vi "Process Outgoing Messages by Frame Type.vi"(0 "J1939 Cluster":T7, 5 "Output Array":T8[](array[typedef]) {"Identifier" format="%08x"}, 7 "Connection Refs":T1, 11 "error in":errorcluster) -> (4 "J1939 Cluster":T7, 13 "Message Errors":errorcluster, 15 "System Error":errorcluster)   [LabVIEW 2013, in "J1939 Addon Engine.lvlib"]
uses:
  Engine/J1939 Addon Engine.lvlib
  J1939 Utilities/Types/CAN Outgoing Message Cluster.ctl
  Types/Setup Information Cluster.ctl
  <vilib>/xnet/xnet.llb/XNET Frame CAN.ctl
  <vilib>/xnet/xnet.llb/XNET Frame Type CAN.ctl
  Types/TP List References.ctl
  Types/BAM Buffer Connections List_Ref.ctl
  Types/Connection Mode Generation Connection Ref.ctl
  Types/BAM Generation Connections List_Ref.ctl
  Types/Address Table Reference.ctl
  Types/RQST Lookup Table Reference.ctl
  Types/TP Connections List State.ctl
  BAM Generation Connections List_Actions.vi
  BAM Generation Create New TP Connection.vi
  Connection Mode Generation Connections List_Actions.vi
  Connection Mode Generation Search for Connection (Local Message).vi
  Connection Mode Generation Create New TP Connection.vi
  J1939 Utilities/Common Conversions.vi
  J1939 Utilities/SubVIs/Convert CAN Arb ID to J1939 ID.vi
  J1939 Utilities/Common Messages.vi
  J1939 Utilities/SubVIs/TP.CM BAM.vi
  J1939 Utilities/SubVIs/TP.DT.vi
  J1939 Utilities/SubVIs/TP.CM RTS.vi
  J1939 Utilities/SubVIs/Convert J1939 ID to CAN Arb ID.vi
  BAM Generation Search for Connection (Local Message).vi
  J1939 Utilities/J1939 Utilities.lvlib
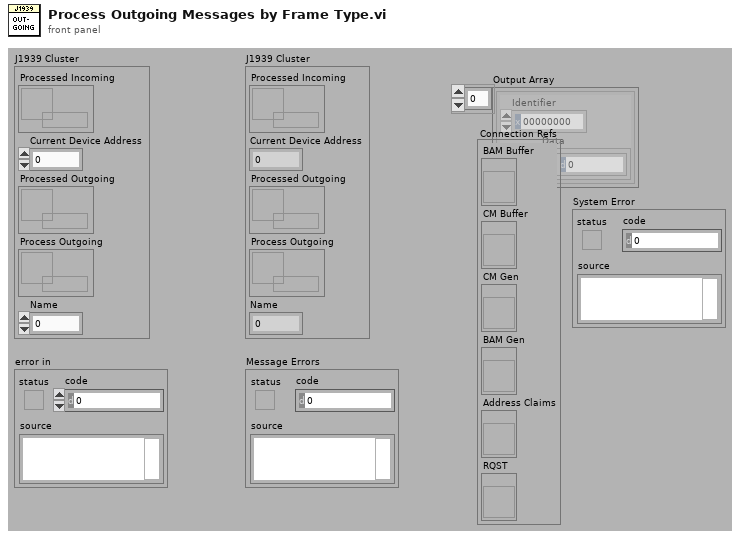
[diagram p1: front panel]
types:
  T1 = typedef "J1939 Addon Engine.lvlib/TP List References.ctl" = cluster{"BAM Buffer":T2, "CM Buffer":T2, "CM Gen":T3, "BAM Gen":T4, "Address Claims":T5, "RQST":T6}
  T2 = typedef "J1939 Addon Engine.lvlib/BAM Buffer Connections List_Ref.ctl" = refnum<vi>
  T3 = typedef "J1939 Addon Engine.lvlib/Connection Mode Generation Connection Ref.ctl" = refnum<vi>
  T4 = typedef "J1939 Addon Engine.lvlib/BAM Generation Connections List_Ref.ctl" = refnum<vi>
  T5 = typedef "J1939 Addon Engine.lvlib/Address Table Reference.ctl" = refnum<vi>
  T6 = typedef "J1939 Addon Engine.lvlib/RQST Lookup Table Reference.ctl" = refnum<vi>
  T7 = typedef "J1939 Addon Engine.lvlib/Setup Information Cluster.ctl" = cluster{"Processed Incoming":refnum<queue>, "Current Device Address":u8, "Processed Outgoing":refnum<queue>, "Process Outgoing":refnum<queue>, "Name":u64}
  T8 = typedef "J1939 Addon Shared.lvlib/J1939 Utilities.lvlib/CAN Outgoing Message Cluster.ctl" = cluster{"Identifier":u32, "Data":u8[]}
  T9 = typedef "J1939 Addon Engine.lvlib/TP Connections List State.ctl" = enum16{"Add", "Update", "Get", "Remove", "Initialize"}
  T10 = typedef "J1939 Addon Shared.lvlib/J1939 Utilities.lvlib/Outgoing Messages Frame Type.ctl" = enum16{"Standard Frame", "BAM", "Connection Mode"}
  T11 = typedef "J1939 Addon Engine.lvlib/BAM Generation Connection Cluster.ctl" = cluster{"Total Packets":u8, "Current Packet to Generate":u8, "Packets":T8[], "Previous Time Stamp":u32, "Total Bytes":u16, "Source Address":u8}
  T12 = typedef "J1939 Addon Engine.lvlib/Connection Mode Generation Connection Cluster.ctl" = cluster{"Total Packets":u8, "Current Packet to Generate":u8, "Packets":T8[], "Previous Time Stamp":u32, "Total Bytes":u16, "Packet Identifier [PDU S + SA]":u16, "Number of Packets to Generate":u8, "PGN":u32}
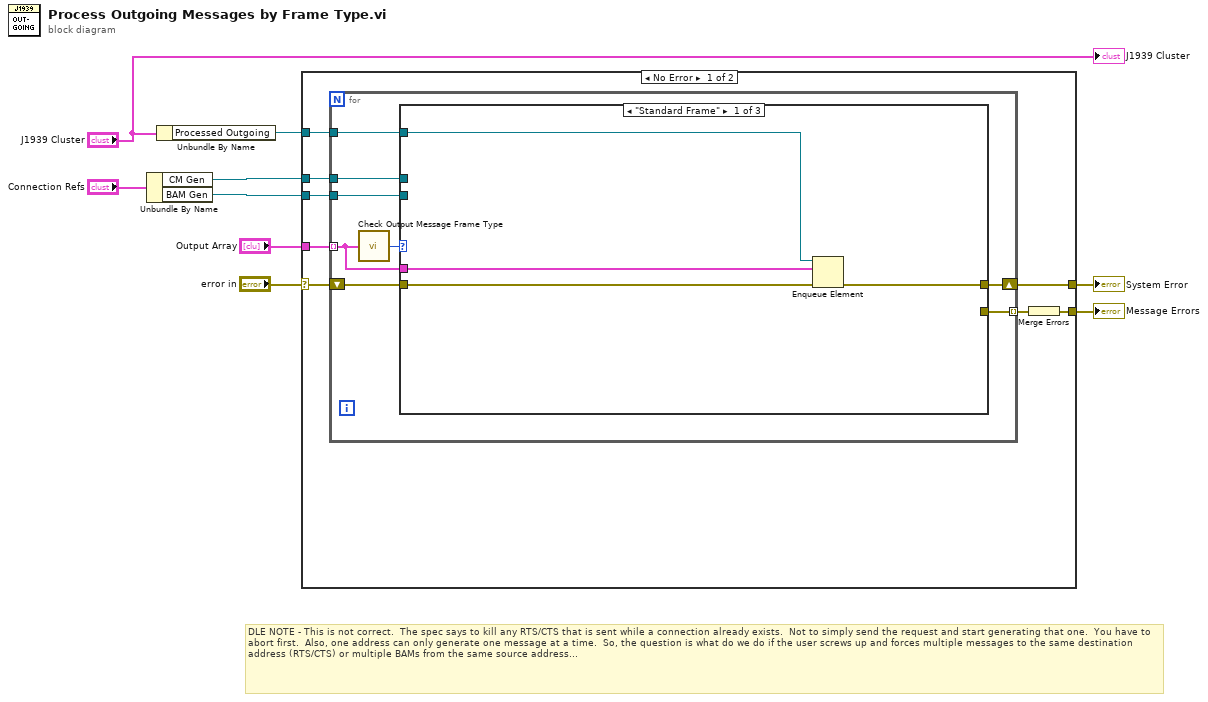
[diagram p0: block diagram]
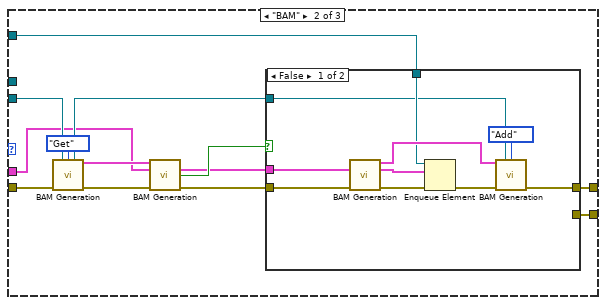
[diagram p2: hidden frame]
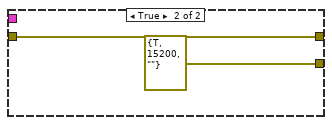
[diagram p3: hidden frame]
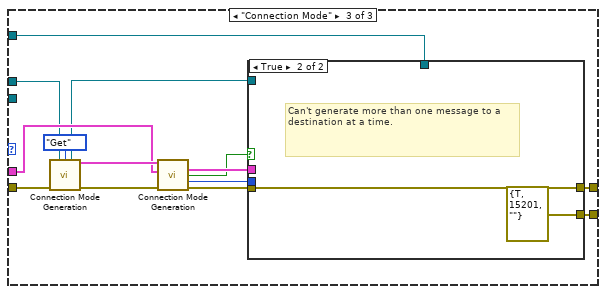
[diagram p4: hidden frame]
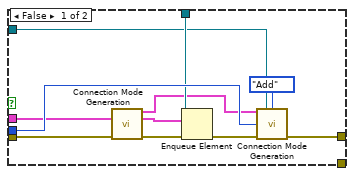
[diagram p5: hidden frame]
diagram:
  # "DLE NOTE - This is not correct.  The spec says to kill any RTS/CTS that is sent while a connection already exists.  Not to simply send the request and start generating that one.  You have to abort first.  Also, one address can only generate one message at a time.  So, the question is what do we do if the user screws up and forces multiple messages to the same destination address (RTS/CTS) or multiple BAMs from the same source address..."
  n1 = Unbundle By Name("Connection Refs") -> ("CM Gen"=w5:T3, "BAM Gen"=w4:T4)
  n2 = Unbundle By Name("J1939 Cluster") -> ("Processed Outgoing"=w9:refnum<queue>)
  n3 = case shown="No Error" "error in" {
    selector: "error in" -> [w14 w82]
    tunnel: w9 -> [w17 _]
    tunnel: "Output Array" -> [w11 _]
    tunnel: w5 -> [w16 _]
    tunnel: w4 -> [w15 _]
    tunnel: [w10 w82] -> w2
    tunnel: [w12 w82] -> w1
    frame No Error {
      n4 = for {
        tunnel: w11 -> [w22] mode=indexing
        tunnel: w17 -> [w24]
        tunnel: w16 -> [w20]
        tunnel: w15 -> [w19]
        tunnel: [w18] -> w13 mode=indexing
        shift-right: [w25] -> w12
        shift-left: w14 -> [w21]
        n5 = call "Check Output Message Frame Type.vi"("Data to Send"=w22) -> ("Frame Type"=w23:T10)  [unwired: 14 out]
        n6 = case shown="\"Standard Frame\"" w23 {
          tunnel: w21 -> [w26 w37 w65]
          tunnel: [w28 w41 w63] -> w25
          tunnel: w24 -> [w29 w42 w61]
          tunnel: w22 -> [w27 w31 w59]
          tunnel: w20 -> [_ _ w58]
          tunnel: w19 -> [_ w35 _]
          tunnel: [_ w32 w55] -> w18
          frame "Standard Frame" {
            n7 = Enqueue Element(queue=w29, element=w27, error in (no error)=w26) -> (error out=w28:errorcluster)  [unwired: 3 out]
          }
          frame "BAM" {
            n8 = call-poly "BAM Generation.vi"("ref in"=w35, "State"=TP_Connections_List_State."Get", "error in (no error)"=w37) -> ("ref out"=w34:T4, "Connections"=w39:T11[], "error out"=w38:errorcluster)  [unwired: 3 in, 7 out]
            n9 = call-poly "BAM Generation.vi"("Connections"=w39, "Data to Send"=w31, "error in (no error)"=w38) -> ("CAN Frame Out"=w30:T8, "Found?"=w33:bool, "error out"=w36:errorcluster)  [unwired: 1 in, 9 out]
            n10 = case shown="False" w33 {
              tunnel: w42 -> [w48 _]
              tunnel: [w47 w53] -> w41
              tunnel: w30 -> [w45 _]
              tunnel: w36 -> [w44 w53]
              tunnel: w34 -> [w43 _]
              tunnel: [_ errorcluster {"status"=TRUE, "code"=15200, "source"=""} ("error out")] -> w32
              frame False {
                n11 = call-poly "BAM Generation.vi"("Data to Send"=w45, "error in (no error)"=w44) -> ("Connection Cluster"=w52:T11, "Connection Management Packet"=w46:T8, "error out"=w50:errorcluster)  [unwired: 3 in, 8 out]
                n12 = Enqueue Element(queue=w48, element=w46, error in (no error)=w50) -> (error out=w51:errorcluster)  [unwired: 3 out]
                n13 = call-poly "BAM Generation.vi"("Connection Cluster"=w52, "ref in"=w43, "State"=TP_Connections_List_State."Add", "error in (no error)"=w51) -> ("error out"=w47:errorcluster)  [unwired: 1 in, 10 out]
              }
              frame True {
              }
            }
          }
          frame "Connection Mode" {
            n14 = call-poly "Connection Mode Generation.vi"("ref in"=w58, "State"=TP_Connections_List_State."Get", "error in (no error)"=w65) -> ("ref out"=w57:T3, "Connections"=w66:T12[], "error out"=w67:errorcluster)  [unwired: 2 in, 8 out]
            n15 = call-poly "Connection Mode Generation.vi"("Connections"=w66, "Data to Send"=w59, "error in (no error)"=w67) -> ("CAN Frame Out"=w60:T8, "Found?"=w56:bool, "Index"=w62:i32, "error out"=w64:errorcluster)  [unwired: 1 in, 8 out]
            n16 = case shown="True" w56 {
              tunnel: w64 -> [w79 w80]
              tunnel: [w78 w80] -> w63
              tunnel: w62 -> [w77 _]
              tunnel: w61 -> [w74 _]
              tunnel: w60 -> [w72 _]
              tunnel: w57 -> [w71 _]
              tunnel: [_ errorcluster {"status"=TRUE, "code"=15201, "source"=""} ("error out")] -> w55
              frame False {
                n17 = call-poly "Connection Mode Generation.vi"("Data to Send"=w72, "error in (no error)"=w79) -> ("Connections Cluster"=w73:T12, "Connection Management Packet"=w70:T8, "error out"=w76:errorcluster)  [unwired: 2 in, 9 out]
                n18 = Enqueue Element(queue=w74, element=w70, error in (no error)=w76) -> (error out=w75:errorcluster)  [unwired: 3 out]
                n19 = call-poly "Connection Mode Generation.vi"("Connection Cluster"=w73, "ref in"=w71, "State"=TP_Connections_List_State."Add" ("f"), "index"=w77, "error in (no error)"=w75) -> ("error out"=w78:errorcluster)  [unwired: 10 out]
              }
              frame True {
                # "Can't generate more than one message to a destination at a time."
              }
            }
          }
        }
      }
      n20 = Merge Errors(w13) -> (w10:errorcluster)
    }
    frame Error {
    }
  }
  "Message Errors" <- w2
  "System Error" <- w1
  "J1939 Cluster" <- "J1939 Cluster"
